vi "SSC Digital Abort.vi"(0 "Digital SSC in":T1[](array[typedef]), 11 "error in":errorcluster) -> (4 "Digital SSC out":T1[](array[typedef]), 15 "error out":errorcluster)   [LabVIEW 2020]
doc: "Stops bursting the pattern on the specified pin(s) or pin group(s)."
uses:
  SSC Digital.ctl
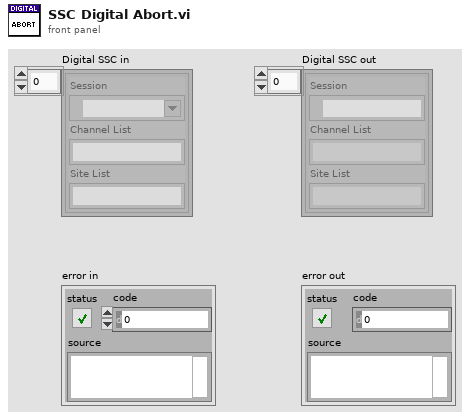
[diagram p1: front panel]
types:
  T1 = typedef "SSC Digital.ctl" = cluster{"Session":refnum<k15>, "Channel List":string, "Site List":string}
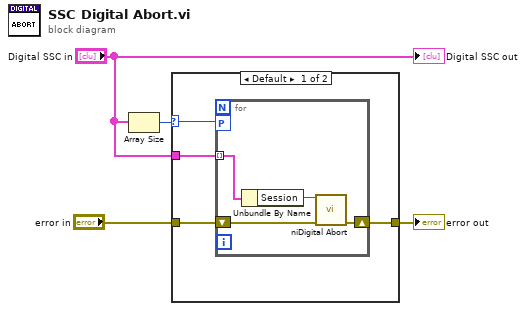
[diagram p0: block diagram]
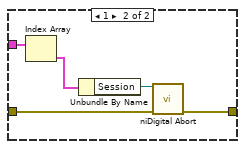
[diagram p2: hidden frame]
diagram:
  n1 = Array Size(array="Digital SSC in") -> (size(s)=w2:i32)
  n2 = case shown="Default" w2 {
    selector: w2 -> [w6 _]
    tunnel: "error in" -> [w8 w17]
    tunnel: [w7 w16] -> w3
    tunnel: "Digital SSC in" -> [w5 w15]
    frame Default {
      n3 = for {
        tunnel: w5 -> [w12] mode=indexing
        workers-P: w6 -> [_]
        shift-right: [w10] -> w7
        shift-left: w8 -> [w11]
        n4 = Unbundle By Name(w12) -> ("Session"=w9:refnum<k15>)
        n5 = call <instrlib>:"niDigital Abort.vi"("instrument handle"=w9, "error in"=w11) -> ("error out"=w10:errorcluster)  [unwired: 12 in, 1 out]
      }
    }
    frame 1 {
      n6 = Index Array(array=w15) -> (element=w13:T1)  [unwired: 1 in]
      n7 = Unbundle By Name(w13) -> ("Session"=w14:refnum<k15>)
      n8 = call <instrlib>:"niDigital Abort.vi"("instrument handle"=w14, "error in"=w17) -> ("error out"=w16:errorcluster)  [unwired: 12 in, 1 out]
    }
  }
  "error out" <- w3
  "Digital SSC out" <- "Digital SSC in"
